vi "Check Action.vi"(6 "HRS Time":dbl, 7 "Values In":dbl[](array[numeric]), 8 "error in (no error)":errorcluster, 11 "Valve in":refnum<class "InterlockControl.lvclass">) -> (0 "error out":errorcluster, 2 "Actions":T1[](array[typedef]), 3 "Valve out":refnum<class "InterlockControl.lvclass">, 5 "Values":dbl[](array[numeric]))   [LabVIEW 2020, in "VolatusControl.lvlib" / "InterlockControl.lvclass"]
uses:
  InterlockControl.lvclass
  Control Action.ctl
  Volatus/MessageQ/MessageQ.lvclass
  Interlock Action.ctl
  InterlockControl.lvclass/InterlockControl.ctl
  lv-vecto/Vecto/Channel DBL/Channel DBL.lvclass/Channel DBL.ctl
  lv-vecto/Vecto/Group DBL/Value by Index.vi
  VolatusControl.lvlib
  lv-vecto/Vecto/Vecto.lvlib
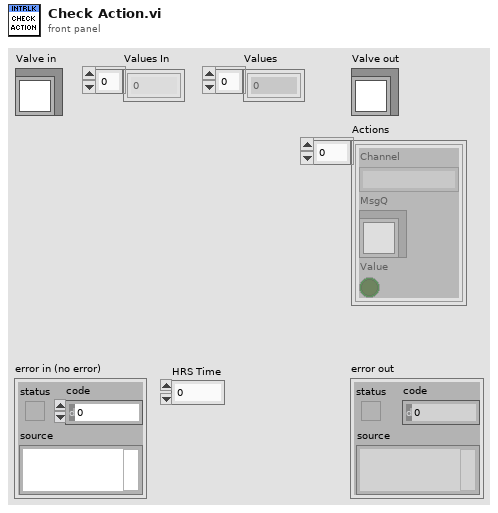
[diagram p1: front panel]
types:
  T1 = typedef "VolatusControl.lvlib/Control Action.ctl" = cluster{"Channel":string, "MsgQ":refnum<class "MessageQ.lvclass">, "Value":bool}
  T2 = typedef "VolatusControl.lvlib/InterlockControl.lvclass/Interlock Action.ctl" = enum16{"None", "Cmd False", "Cmd True"}
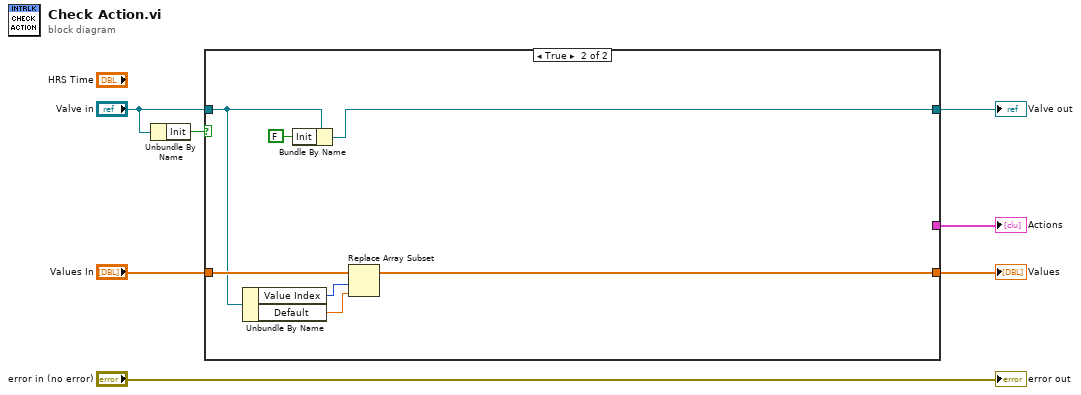
[diagram p0: block diagram]
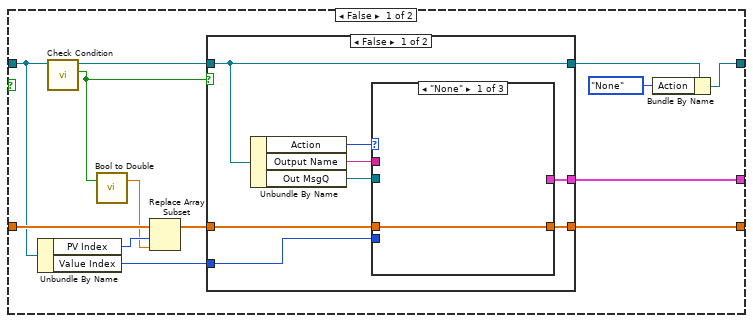
[diagram p2: hidden frame]
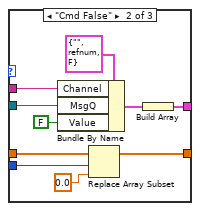
[diagram p3: hidden frame]
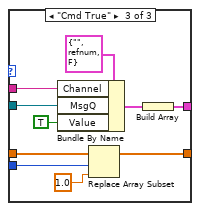
[diagram p4: hidden frame]
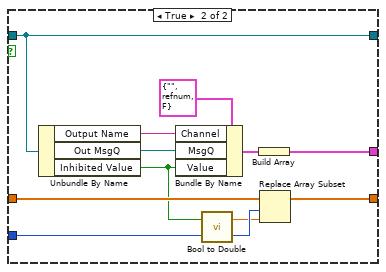
[diagram p5: hidden frame]
diagram:
  n1 = Unbundle By Name("Valve in") -> ("Init"=w1:bool)
  n2 = case shown="True" w1 {
    tunnel: "Values In" -> [w20 w67]
    tunnel: [w19 _] -> w5
    tunnel: [w18 w66] -> w4
    tunnel: [w17 w62] -> w3
    tunnel: "Valve in" -> [w8 w65]
    frame False {
      n3 = Unbundle By Name(w8) -> ("PV Index"=w12:i32, "Value Index"=w9:i32)
      n4 = call "Check Condition.vi"("InterlockControl in"=w8) -> ("Interlocked"=w13:bool, "InterlockControl out"=w15:refnum<class "InterlockControl.lvclass">)  [unwired: 8 in, 1 out]
      n5 = call "Bool to Double.vi"("Bool"=w13) -> ("Double"=w11:dbl)  [unwired: 2 in]
      n6 = Replace Array Subset(array=w20, new element=w11, index=w12) -> (w10:dbl[])
      n7 = case shown="False" w13 {
        tunnel: w15 -> [w28 w57]
        tunnel: [w28 w57] -> w14
        tunnel: [w24 w55] -> w19
        tunnel: w10 -> [w23 w54]
        tunnel: w9 -> [w22 w52]
        tunnel: [w21 w53] -> w18
        frame False {
          n8 = Unbundle By Name(w28) -> ("Action"=w27:T2, "Output Name"=w26:string, "Out MsgQ"=w25:refnum<class "MessageQ.lvclass">)
          n9 = case shown="\"None\"" w27 {
            tunnel: w26 -> [_ w38 w48]
            tunnel: w25 -> [_ w37 w47]
            tunnel: [_ w34 w44] -> w24
            tunnel: w23 -> [w29 w32 w42]
            tunnel: w22 -> [_ w30 w43]
            tunnel: [w29 w31 w40] -> w21
            frame "None" {
            }
            frame "Cmd False" {
              n10 = Bundle By Name(cluster=T1 {"Channel"="", "MsgQ"=refnum, "Value"=FALSE} ("Action"), "Channel"=w38, "MsgQ"=w37, "Value"=FALSE) -> (w36:T1)
              n11 = Replace Array Subset(array=w32, new element=0.0 ("new element/subarray"), index=w30) -> (w31:dbl[])
              n12 = Build Array(w36) -> (w34:T1[])
            }
            frame "Cmd True" {
              n13 = Bundle By Name(cluster=T1 {"Channel"="", "MsgQ"=refnum, "Value"=FALSE} ("Action"), "Channel"=w48, "MsgQ"=w47, "Value"=TRUE) -> (w46:T1)
              n14 = Replace Array Subset(array=w42, new element=1.0 ("new element/subarray"), index=w43) -> (w40:dbl[])
              n15 = Build Array(w46) -> (w44:T1[])
            }
          }
        }
        frame True {
          n16 = Unbundle By Name(w57) -> ("Output Name"=w59:string, "Out MsgQ"=w58:refnum<class "MessageQ.lvclass">, "Inhibited Value"=w50:bool)
          n17 = Bundle By Name(cluster=T1 {"Channel"="", "MsgQ"=refnum, "Value"=FALSE} ("Action"), "Channel"=w59, "MsgQ"=w58, "Value"=w50) -> (w56:T1)
          n18 = call "Bool to Double.vi"("Bool"=w50) -> ("Double"=w51:dbl)  [unwired: 2 in]
          n19 = Build Array(w56) -> (w55:T1[])
          n20 = Replace Array Subset(array=w54, new element=w51, index=w52) -> (w53:dbl[])
        }
      }
      n21 = Bundle By Name(cluster=w14, "Action"=Interlock_Action."None") -> (w17:refnum<class "InterlockControl.lvclass">)
    }
    frame True {
      n22 = Unbundle By Name(w65) -> ("Value Index"=w64:i32, "Default"=w63:dbl)
      n23 = Bundle By Name(cluster=w65, "Init"=FALSE) -> (w62:refnum<class "InterlockControl.lvclass">)
      n24 = Replace Array Subset(array=w67, new element=w63, index=w64) -> (w66:dbl[])
    }
  }
  "Valve out" <- w3
  "Actions" <- w5
  "Values" <- w4
  "error out" <- "error in (no error)"
